vi "AddControl_Core.vi"(8 "error in (no error)":errorcluster, 9 "CtlRef":refnum<vi>, 10 "CtlName":string, 11 "ctlrRef_VAT in":refnum<class "ctlRef_VAT.lvclass">) -> (0 "error out":errorcluster, 3 "ctlrRef_VAT out":refnum<class "ctlRef_VAT.lvclass">)   [LabVIEW 2020, in "CtlReferences.lvlib" / "ctlRef_VAT.lvclass"]
uses:
  ctlRef_VAT.lvclass
  ctlRef_VAT.lvclass/ctlRef_VAT.ctl
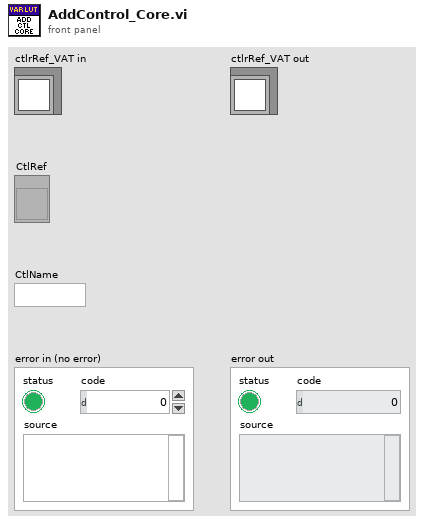
[diagram p1: front panel]
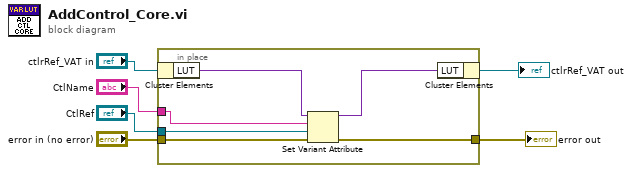
[diagram p0: block diagram]
diagram:
  n1 = in-place {
    in-place-border: "CtlRef" -> [w9]
    in-place-border: [w10] -> w1
    in-place-border: "error in (no error)" -> [w8]
    in-place-border: "CtlName" -> [w7]
    n2 = in-place-cluster #1("ctlrRef_VAT in") -> ("LUT"=w12:variant)
    n3 = Set Variant Attribute(Variant=w12, name=w7, value=w9, error in=w8) -> (Variant out=w11:variant, error out=w10:errorcluster)  [unwired: 1 out]
    n4 = in-place-cluster #1("LUT"=w11) -> (→"ctlrRef_VAT out":refnum<class "ctlRef_VAT.lvclass">)
  }
  "error out" <- w1
